vi "q5 even odd counts.vi"() -> ()   [LabVIEW 2025]
panel:
  out "odd":i32
  out "even":i32
  in  "Array":dbl[](array[numeric])
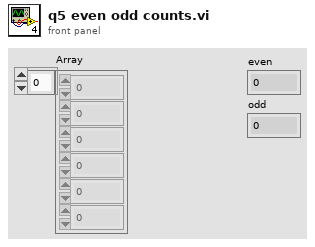
[diagram p1: front panel]
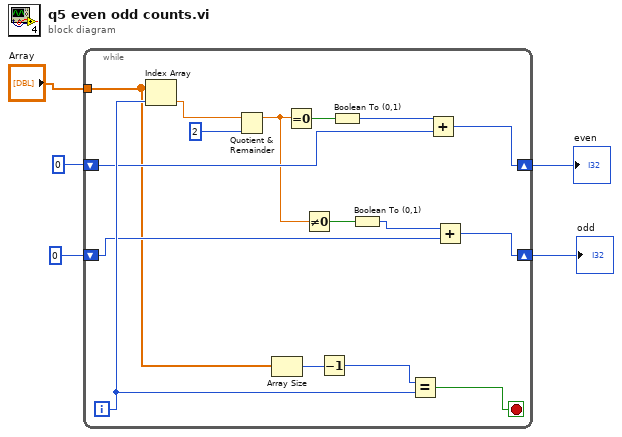
[diagram p0: block diagram]
diagram:
  n1 = while {
    tunnel: "Array" -> [w6]
    shift-right: [w12] -> w3
    shift-left: 0 -> [w13]
    shift-right: [w7] -> w1
    shift-left: 0 -> [w8]
    i -> [w18]
    stop <- w21 stop-if-true
    n2 = Index Array(array=w6, index=w18) -> (element=w17:dbl)
    n3 = Quotient & Remainder(x=w17, y=2) -> (x-y*floor(x/y)=w11:dbl)  [unwired: 1 out]
    n4 = Array Size(array=w6) -> (size(s)=w20:i32)
    n5 = Equal To 0?(x=w11) -> (x = 0?=w15:bool)
    n6 = Not Equal To 0?(x=w11) -> (x != 0?=w10:bool)
    n7 = Decrement(x=w20) -> (x-1=w19:i32)
    n8 = Boolean To (0,1)(Boolean=w15) -> (0, 1=w14:i16)
    n9 = Boolean To (0,1)(Boolean=w10) -> (0, 1=w9:i16)
    n10 = Equal?(x=w19, y=w18) -> (x = y?=w21:bool)
    n11 = Add(x=w14, y=w13) -> (x+y=w12:i32)
    n12 = Add(x=w9, y=w8) -> (x+y=w7:i32)
  }
  "even" <- w3
  "odd" <- w1
